vi "proc_peek_stdout.vi"(8 "error in":errorcluster, 10 "size":i32, 11 "process instance handle in":u32[](array[numeric])) -> (0 "error out":errorcluster, 1 "bytes read":i32, 2 "read buffer":string, 3 "process instance handle out":u32[](array[numeric]), 4 "exited":bool, 5 "bytes to read":i32)   [LabVIEW 2012]
doc: "Peeks process instance stdout pipe. Returnes array of bytes terminated with '\\0', remaining bytes count in pipe, process status."
panel:
  in  "toread mem":i32
  in  "read mem":i32
  in  "exit mem":i32
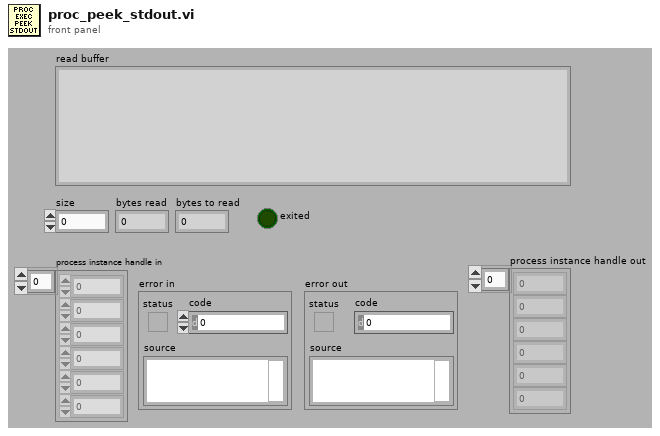
[diagram p1: front panel]
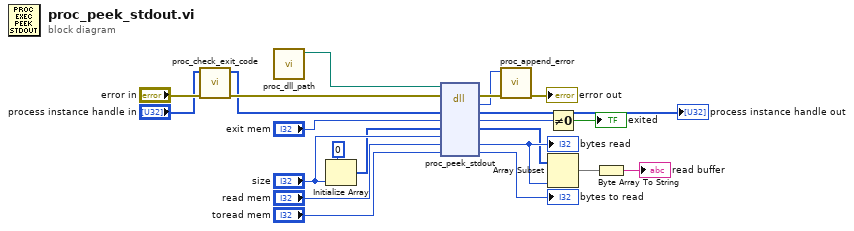
[diagram p0: block diagram]
diagram:
  n1 = call "proc_check_exit_code.vi"("error in"="error in", "instance handle in"="process instance handle in") -> ("error out"=w3:errorcluster, "instance handle out"=w1:u32[])  [unwired: 5 in, 3 out]
  n2 = call "proc_dll_path.vi"() -> ("path out"=w22:path)  [unwired: 10 in, 1 out]
  n3 = Initialize Array(u8 0 ("element"), "size") -> (w17:u8[])
  n4 = dll-call lib="lv_proc.dll" fn="proc_peek_stdout"(path in=w22, error in=w3, "proc"=w1, "exit"="exit mem", "buffer"=w17, "size"="size", "read"="read mem", "toread"="toread mem") -> (error out=w7:errorcluster, "error"=w5:i32, "proc"=→"process instance handle out":u32[], "exit"=w12:i32, "buffer"=w10:u8[], "read"=w15:i32, "toread"=→"bytes to read":i32)  [unwired: 2 in, 1 out]
  "bytes read" <- w15
  n5 = call "proc_append_error.vi"("error in"=w7, "code in"=w5) -> ("error out"=→"error out":errorcluster)  [unwired: 8 in, 1 out]
  n6 = Not Equal To 0?(x=w12) -> (x != 0?=→"exited":bool)
  n7 = Array Subset(array=w10, length=w15) -> (w9:u8[])  [unwired: 1 in]
  n8 = Byte Array To String(unsigned byte array=w9) -> (string=→"read buffer":string)
